vi "getDescription.vi"(8 "error in (no error)":errorcluster, 11 "Soy in":refnum<class "Soy.lvclass">) -> (0 "error out":errorcluster, 2 "description":string, 3 "Soy out":refnum<class "Soy.lvclass">)   [LabVIEW 2017, in "Soy.lvclass"]
uses:
  Soy.lvclass
  CondimentDecorator/CondimentDecorator.lvclass
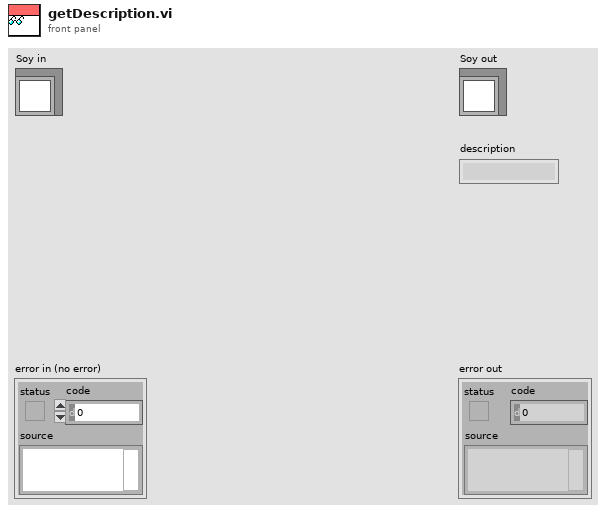
[diagram p1: front panel]
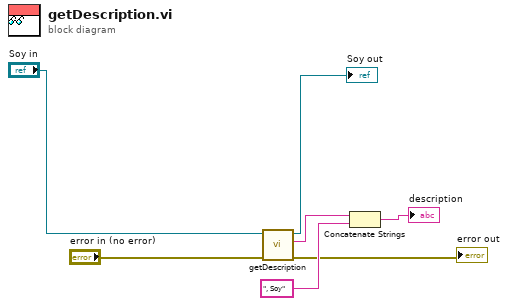
[diagram p0: block diagram]
diagram:
  n1 = call-parent "getDescription.vi"("error in (no error)"="error in (no error)", "CondimentDecorator in"="Soy in") -> ("error out"=→"error out":errorcluster, "description"=w1:string, "CondimentDecorator out"=→"Soy out":refnum<class "Soy.lvclass">)  [unwired: 7 in]
  n2 = Concatenate Strings(w1, ", Soy") -> (→"description":string)
